vi "Teleop.vi"(10 "Match Info":T1={"Autonomous Elapsed Seconds"=0.0, "TeleOp Elapsed Seconds"=0.0, "Disabled Elapsed Seconds"=0.0, "Visited Autonomous"=FALSE, "Visited TeleOp"=FALSE, "Visited Disabled"=FALSE, "Autonomous Settings"={"Autonomous Style"=enum."Independent", "VI Refnum"=refnum}}, 11 "Call Context":T2) -> ()   [LabVIEW 2014]
doc: "This VI is called for each TeleOp packet received from the DS where the robot is not disabled. It is often used to read from the joysticks and update I/O or to update setpoints for timed control loops. It should complete and return within 20 milliseconds or it may miss DS packets."
uses:
  <vilib>/Rock Robotics/WPI/DriverStation/WPI_DriverStationDerivedRobotMode.ctl
  <vilib>/Rock Robotics/WPI/DriverStation/WPI_DriverStationMatch Info.ctl
  <vilib>/Rock Robotics/WPI/RobotDrive/WPI_RobotDriveGetSetRefNum.vi
  <vilib>/Rock Robotics/WPI/Joystick/WPI_JoystickGetSetRefNum.vi
  Robot Global Data.vi
  <vilib>/Rock Robotics/Network Tables/SD Write Boolean Array.vi
  <vilib>/Rock Robotics/Network Tables/SD Write Numeric Array.vi
  <vilib>/Rock Robotics/Network Tables/SD Read Number.vi
  <vilib>/Rock Robotics/Network Tables/SD Write Number.vi
  <vilib>/Rock Robotics/Network Tables/SD Write Boolean.vi
  <vilib>/Rock Robotics/WPI/RobotDrive/WPI_RobotDriveMecanumDrive_Cartesian.vi
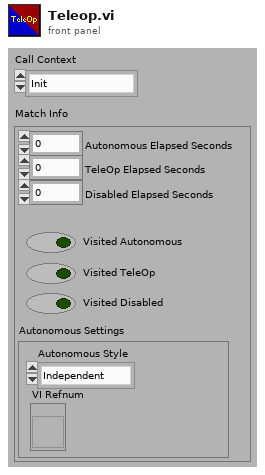
[diagram p1: front panel]
types:
  T1 = typedef "WPI_DriverStationMatch Info.ctl" = cluster{"Autonomous Elapsed Seconds":dbl, "TeleOp Elapsed Seconds":dbl, "Disabled Elapsed Seconds":dbl, "Visited Autonomous":bool, "Visited TeleOp":bool, "Visited Disabled":bool, "Autonomous Settings":cluster{"Autonomous Style":enum16{"Iterative", "Independent"}, "VI Refnum":refnum<vi>}}
  T2 = typedef "WPI_DriverStationDerivedRobotMode.ctl" = enum16{"Init", "Execute", "Stop"}
  T3 = typedef "WPI_RobotDriveDevRef.ctl" = cluster{"DevStatus":errorcluster, "Motors[]":T4[], "Square Inputs":bool, "Max Output":dbl}
  T4 = typedef "WPI_MotorControlDeviceRef.ctl" = cluster{"DeviceStatus":errorcluster, "Type":T5, "PWM":cluster{"Controller":T6, "PWM Channel":T7, "DeadBand":T8}, "CAN":cluster{"Device Number":u8, "Control Mode":T9, "Semaphore":T10, "Max Vout":dbl, "TalonSRX Control Mode":T11}, "Invert":bool, "TransformRef":T12, "InvTransformRef":T12}
  T5 = typedef "WPI_MotorControlType.ctl" = enum16{"PWM", "CAN", "CANTalonSRX"}
  T6 = typedef "FPGA_TypedefDigitalModule.ctl" = enum16{"Controller 1"}
  T7 = typedef "FPGA_DIOPWMChannel.ctl" = enum8{"PWM 0", "PWM 1", "PWM 2", "PWM 3", "PWM 4", "PWM 5", "PWM 6", "PWM 7", "PWM 8", "PWM 9", "PWM MXP 0", "PWM MXP 1", "PWM MXP 2", "PWM MXP 3", "PWM MXP 4", "PWM MXP 5", "PWM MXP 6", "PWM MXP 7", "PWM MXP 8", "PWM MXP 9", "Invalid"}
  T8 = typedef "WPI_PWMDeadband.ctl" = cluster{"Name":string, "maxPositivePwm":i32, "minPositivePwm":i32, "centerPwm":i32, "maxNegativePwm":i32, "minNegativePwm":i32, "angularRange":u16}
  T9 = typedef "WPI_CANJaguar_ControlMode.ctl" = enum8{"Percent VBus", "Current", "Speed", "Position", "Voltage"}
  T10 = typedef "Semaphore RefNum" = refnum<k1>
  T11 = typedef "WPI_CANTalonSRX_APIControlMode.ctl" = enum8{"Percent VBus", "Speed", "Position", "Slave", "Unchanged / Invalid"}
  T12 = typedef "WPI_PWMTransform_ConPane.ctl" = refnum<vi>
  T13 = typedef "WPI_JoystickDevRef.ctl" = cluster{"Device":T14}
  T14 = typedef "WPI_JoystickDeviceEnum.ctl" = enum16{"USB 0", "USB 1", "USB 2", "USB 3", "USB 4", "USB 5"}
  T15 = typedef "WPI_EncoderDevRef.ctl" = cluster{"DevStatus":errorcluster, "EncoderIndex":T16, "CounterIndex":T17, "DistancePerCount":dbl, "Decoding Type":T18}
  T16 = typedef "FPGA_EncoderIdx.ctl" = enum8{"Enc 0", "Enc 1", "Enc 2", "Enc 3", "Enc 4", "Enc 5", "Enc 6", "Enc 7", "Invalid"}
  T17 = typedef "FPGA_CounterCtrSystemIndex.ctl" = enum8{"Ctr 0", "Ctr 1", "Ctr 2", "Ctr 3", "Ctr 4", "Ctr 5", "Ctr 6", "Ctr 7", "Invalid"}
  T18 = typedef "WPI_EncoderType.ctl" = enum16{"1x", "2x", "4x"}
  T19 = typedef "WPI_GyroDevRef.ctl" = cluster{"DevStatus":errorcluster, "Analog Module":T20, "Analog Channel":T21, "Offset":dbl, "Gain (VoltsPerDegree/Second)":dbl}
  T20 = typedef "FPGA_TypedefAnalogModule.ctl" = enum16{"Controller 1"}
  T21 = typedef "FPGA_AIChannel.ctl" = enum8{"AI 0", "AI 1", "AI 2", "AI 3", "AI MXP 0", "AI MXP 1", "AI MXP 2", "AI MXP 3", "Invalid"}
  T22 = typedef "WPI_DigitalInputDevRef.ctl" = cluster{"DevStatus":errorcluster, "DIO Channel":T23, "Controller":T6}
  T23 = typedef "FPGA_DIOChannel.ctl" = enum8{"DIO 0", "DIO 1", "DIO 2", "DIO 3", "DIO 4", "DIO 5", "DIO 6", "DIO 7", "DIO 8", "DIO 9", "DIO MXP 0", "DIO MXP 1", "DIO MXP 2", "DIO MXP 3", "DIO MXP 4", "DIO MXP 5", "DIO MXP 6", "DIO MXP 7", "DIO MXP 8", "DIO MXP 9", "DIO MXP 10", "DIO MXP 11", "DIO MXP 12", "DIO MXP 13", "DIO MXP 14", "DIO MXP 15", "Invalid"}
  T24 = enum16{"Start", "Extending", "Lowering", "Grabbing", "Lifting", "Holding", "Placing", "Opening", "Dropping", "Score", "Exit", "Manual"}
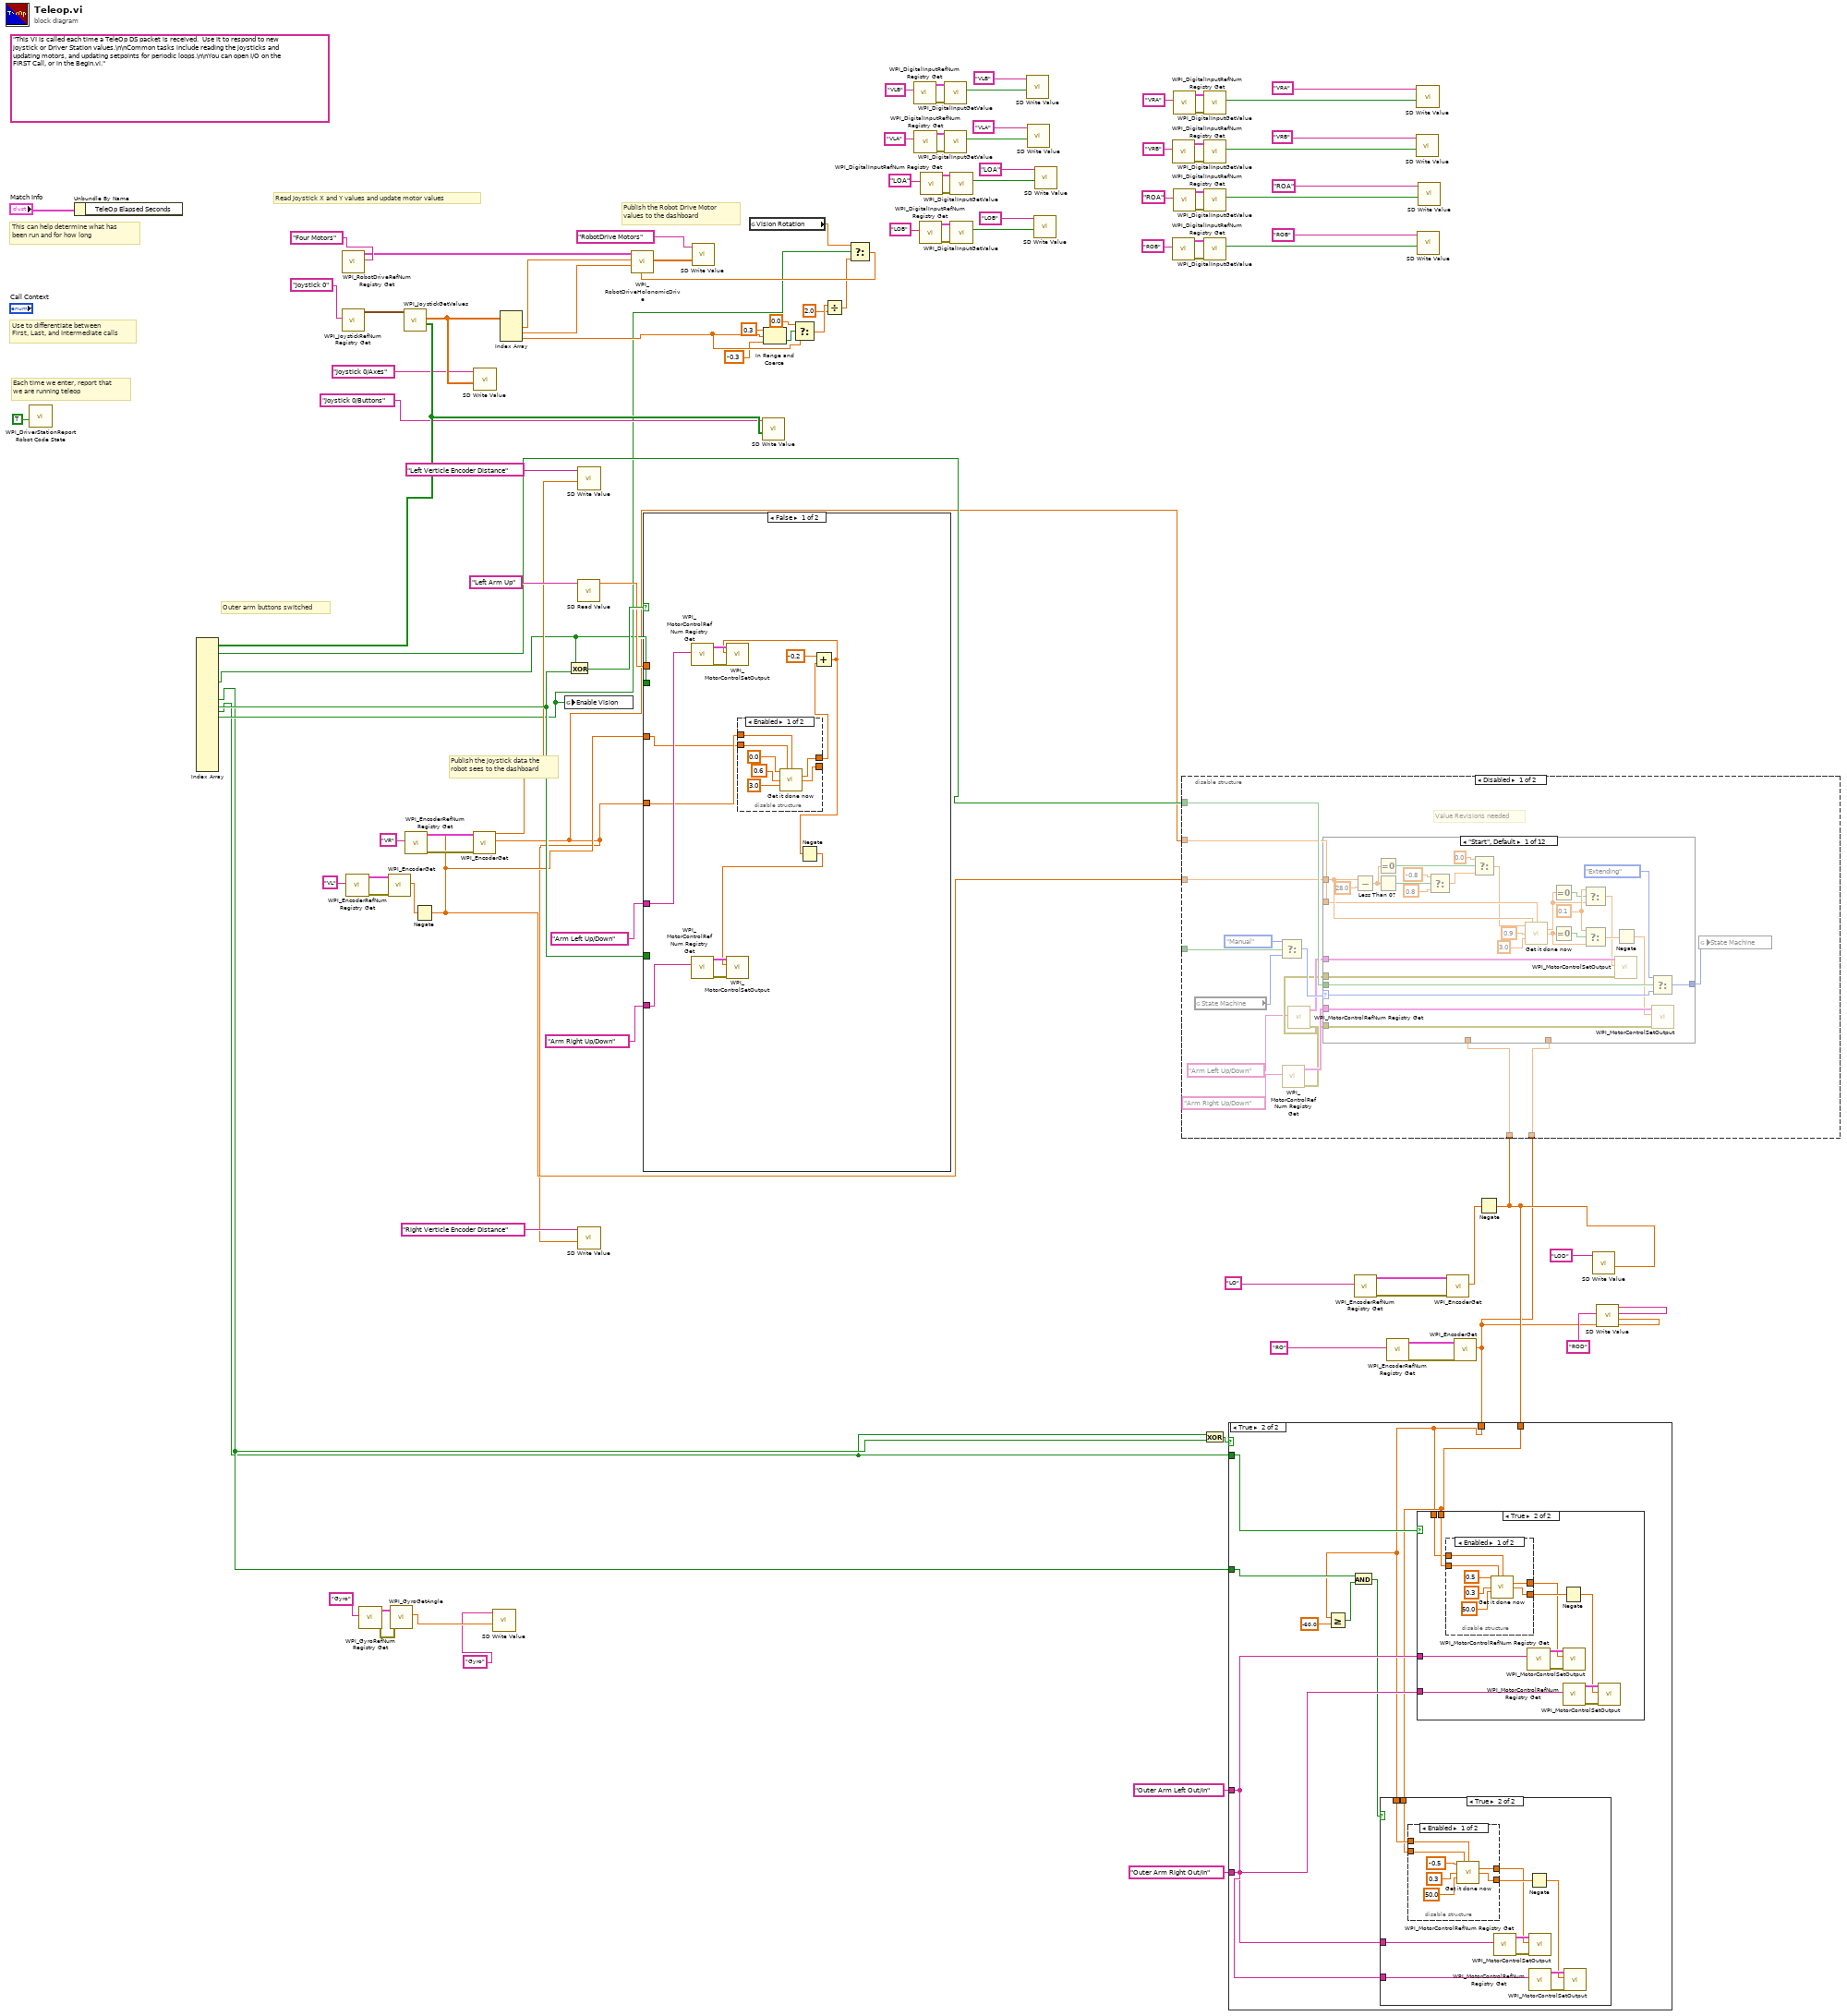
[diagram p0: block diagram]
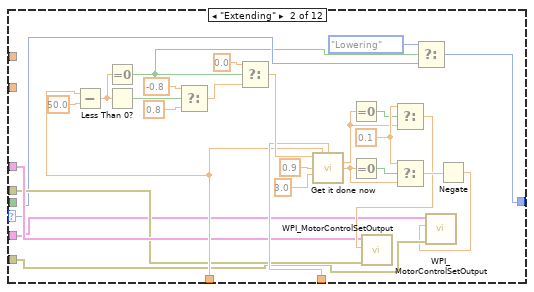
[diagram p2: hidden frame]
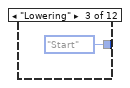
[diagram p3: hidden frame]
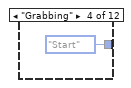
[diagram p4: hidden frame]
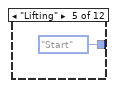
[diagram p5: hidden frame]
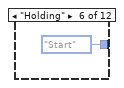
[diagram p6: hidden frame]
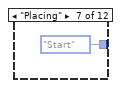
[diagram p7: hidden frame]
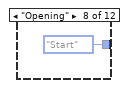
[diagram p8: hidden frame]
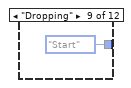
[diagram p9: hidden frame]
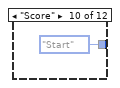
[diagram p10: hidden frame]
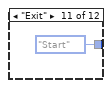
[diagram p11: hidden frame]
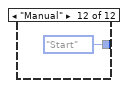
[diagram p12: hidden frame]
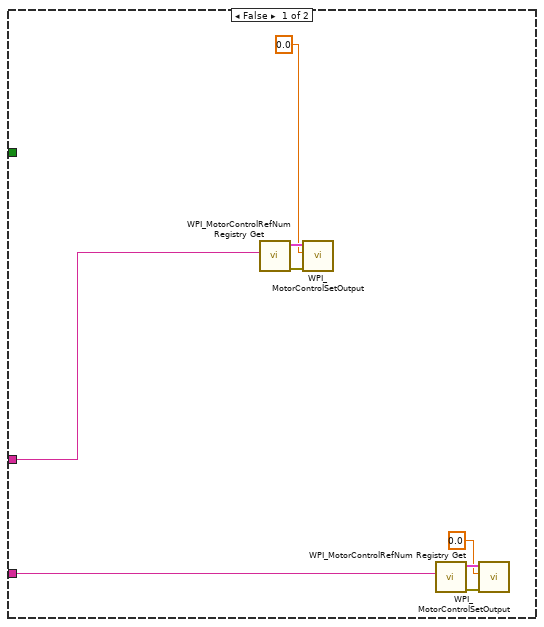
[diagram p14: hidden frame]
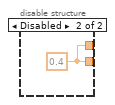
[diagram p16: hidden frame]
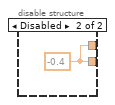
[diagram p18: hidden frame]
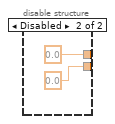
[diagram p19: hidden frame]
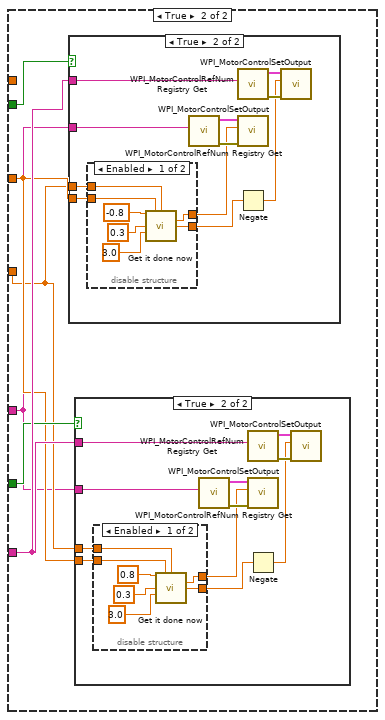
[diagram p20: hidden frame]
diagram:
  w6 = "ROD" ("Name")
  (unwired) "This VI is called each time a TeleOp DS packet is received.  Use it to respond to new joystick or Driver Station values.\n\nCommon tasks include reading the joysticks and updating motors, and updating setpoints for periodic loops.\n\nYou can open I/O on the FIRST Call, or in the Begin.vi."
  # "Outer arm buttons switched"
  # "Publish the joystick data the\nrobot sees to the dashboard"
  # "Publish the Robot Drive Motor\nvalues to the dashboard"
  # "Each time we enter, report that\nwe are running teleop"
  # "Use to differentiate between\nFirst, Last, and Intermediate calls"
  # "This can help determine what has\nbeen run and for how long"
  # "Read Joystick X and Y values and update motor values"
  n1 = call <vilib>:"WPI_DriverStationReport Robot Code State.vi"("TeleOp"=TRUE ("Autonomous")) -> ()  [unwired: 10 in, 1 out]
  n2 = Unbundle By Name("Match Info") -> ()  [unwired: 1 out]
  n3 = call <vilib>:"WPI_RobotDriveRefNum Registry Get.vi"("refnum name"="Four Motors") -> ("RobotDriveDevRef"=w103:T3)  [unwired: 1 in, 9 out]
  n4 = call <vilib>:"WPI_JoystickRefNum Registry Get.vi"("refnum name"="Joystick 0") -> ("JoystickDevRef"=w101:T13)  [unwired: 1 in, 9 out]
  n5 = call <vilib>:"WPI_EncoderRefNum Registry Get.vi"("refnum name"="VL") -> ("error out"=w80:errorcluster, "EncoderDevRef"=w81:T15)  [unwired: 9 in]
  n6 = call <vilib>:"WPI_GyroRefNum Registry Get.vi"("refnum name"="Gyro") -> ("error out"=w69:errorcluster, "GyroDevRef"=w68:T19)  [unwired: 9 in]
  n7 = call <vilib>:"WPI_EncoderGet.vi"("error in (no error)"=w80, "EncoderDevRef"=w81) -> ("Distance"=w62:dbl)  [unwired: 4 in, 5 out]
  n8 = call <vilib>:"WPI_GyroGetAngle.vi"("error in (no error)"=w69, "GyroDevRef"=w68) -> ("Angle"=w66:dbl)  [unwired: 6 in, 3 out]
  n9 = call <vilib>:"WPI_JoystickGetValues.vi"("JoystickDevRef"=w101) -> ("Buttons"=w96:bool[], "Axes"=w97:dbl[])  [unwired: 6 in, 3 out]
  n10 = Index Array(array=w96) -> (element #1=w11:bool, element #4=w90:bool, element #6=w8:bool, element #9=w4:bool, element #11=w3:bool, element #12=w9:bool)  [unwired: 21 in, 15 out]
  n11 = call <vilib>:"WPI_EncoderRefNum Registry Get.vi"("refnum name"="VR") -> ("error out"=w84:errorcluster, "EncoderDevRef"=w83:T15)  [unwired: 9 in]
  n12 = Negate(x=w62) -> (-x=w10:dbl)
  n13 = call <vilib>:"WPI_EncoderGet.vi"("error in (no error)"=w84, "EncoderDevRef"=w83) -> ("Distance"=w1:dbl)  [unwired: 4 in, 5 out]
  n14 = call-poly <vilib>:"SD Write Value.vi"("Numeric Array"=w97, "Name"="Joystick 0/Axes") -> ()  [unwired: 8 in, 2 out]
  n15 = call-poly <vilib>:"SD Write Value.vi"("Numeric"=w66, "Name"="Gyro") -> ()  [unwired: 8 in, 2 out]
  n16 = Index Array(array=w97) -> (element #1=w95:dbl, element #2=w94:dbl, element #3=w72:dbl)  [unwired: 3 in]
  n17 = global write "Robot Global Data.vi" "Enable Vision"(w9) -> ()
  n18 = Exclusive Or(1:w90, 2:w8) -> (0:w91:bool)
  n19 = call-poly <vilib>:"SD Read Value.vi"("Name"="Left Arm Up") -> ("Numeric"=w86:dbl)  [unwired: 8 in, 2 out]
  n20 = call-poly <vilib>:"SD Write Value.vi"("Numeric"=w10, "Name"="Left Verticle Encoder Distance") -> ()  [unwired: 8 in, 2 out]
  n21 = call-poly <vilib>:"SD Write Value.vi"("Numeric"=w1, "Name"="Right Verticle Encoder Distance") -> ()  [unwired: 8 in, 2 out]
  n22 = case shown="False" w91 {
    tunnel: w8 -> [_ w127]
    tunnel: w90 -> [_ w131]
    tunnel: "Arm Left Up/Down" ("refnum name") -> [w113 w128]
    tunnel: "Arm Right Up/Down" ("refnum name") -> [w112 w132]
    tunnel: w86 -> [_ _]
    tunnel: w1 -> [w111 w129]
    tunnel: w10 -> [w110 w130]
    frame False {
      n23 = call <vilib>:"WPI_MotorControlRefNum Registry Get.vi"("refnum name"=w113) -> ("error out"=w116:errorcluster, "MotorControlDevRef"=w117:T4)  [unwired: 9 in]
      n24 = call <vilib>:"WPI_MotorControlRefNum Registry Get.vi"("refnum name"=w112) -> ("error out"=w114:errorcluster, "MotorControlDevRef"=w115:T4)  [unwired: 9 in]
      n25 = disable-structure shown="Enabled" {
        disable-tunnel: w111 -> [w122 _]
        disable-tunnel: w110 -> [w121 _]
        disable-tunnel: [w123 0.0 ("Output")] -> _
        disable-tunnel: [w124 0.0 ("Output")] -> w109
        frame Enabled {
          n26 = call "Get it done now.vi"("Joystick Command"=0.0, "Encoder 0 Distance"=w121, "Encoder 1 Distance"=w122, "Maximum PWM Change"=0.6, "Max Following Error"=3.0) -> ("Motor 0 Command"=w124:dbl, "Motor 1 Command"=w123:dbl)  [unwired: 7 in, 2 out]
        }
        frame Disabled {
        }
      }
      n27 = Add(x=-0.2, y=w109) -> (x+y=w107:dbl)
      n28 = call <vilib>:"WPI_MotorControlSetOutput.vi"("error in (no error)"=w116, "Output"=w107, "MotorControlDevRef"=w117) -> ()  [unwired: 6 in, 3 out]
      n29 = Negate(x=w107) -> (-x=w106:dbl)
      n30 = call <vilib>:"WPI_MotorControlSetOutput.vi"("error in (no error)"=w114, "Output"=w106, "MotorControlDevRef"=w115) -> ()  [unwired: 6 in, 3 out]
    }
    frame True {
      n31 = case shown="True" w127 {
        tunnel: w128 -> [_ w139]
        tunnel: w132 -> [_ w133]
        tunnel: w129 -> [_ w138]
        tunnel: w130 -> [_ w137]
        frame False {
        }
        frame True {
          n32 = disable-structure shown="Enabled" {
            disable-tunnel: w138 -> [w150 _]
            disable-tunnel: w137 -> [w149 _]
            disable-tunnel: [w144 w151] -> w136
            disable-tunnel: [w145 w151] -> w134
            frame Enabled {
              n33 = call "Get it done now.vi"("Joystick Command"=-0.8 ("Maximum PWM Change"), "Encoder 0 Distance"=w149, "Encoder 1 Distance"=w150, "Maximum PWM Change"=0.3, "Max Following Error"=3.0) -> ("Motor 0 Command"=w145:dbl, "Motor 1 Command"=w144:dbl)  [unwired: 7 in, 2 out]
            }
            frame Disabled {
              w151 = 0.3 ("Motor 1 Command")
            }
          }
          n34 = call <vilib>:"WPI_MotorControlRefNum Registry Get.vi"("refnum name"=w139) -> ("error out"=w143:errorcluster, "MotorControlDevRef"=w142:T4)  [unwired: 9 in]
          n35 = call <vilib>:"WPI_MotorControlRefNum Registry Get.vi"("refnum name"=w133) -> ("error out"=w141:errorcluster, "MotorControlDevRef"=w140:T4)  [unwired: 9 in]
          n36 = call <vilib>:"WPI_MotorControlSetOutput.vi"("error in (no error)"=w143, "Output"=w134, "MotorControlDevRef"=w142) -> ()  [unwired: 6 in, 3 out]
          n37 = Negate(x=w136) -> (-x=w135:dbl)
          n38 = call <vilib>:"WPI_MotorControlSetOutput.vi"("error in (no error)"=w141, "Output"=w135, "MotorControlDevRef"=w140) -> ()  [unwired: 6 in, 3 out]
        }
      }
      n39 = case shown="True" w131 {
        tunnel: w128 -> [_ w158]
        tunnel: w132 -> [_ w157]
        tunnel: w130 -> [_ w156]
        tunnel: w129 -> [_ w155]
        frame False {
        }
        frame True {
          n40 = disable-structure shown="Enabled" {
            disable-tunnel: w156 -> [w166 _]
            disable-tunnel: w155 -> [w167 _]
            disable-tunnel: [w168 w170] -> w154
            disable-tunnel: [w169 w170] -> w152
            frame Enabled {
              n41 = call "Get it done now.vi"("Joystick Command"=0.8 ("Maximum PWM Change"), "Encoder 0 Distance"=w166, "Encoder 1 Distance"=w167, "Maximum PWM Change"=0.3, "Max Following Error"=3.0) -> ("Motor 0 Command"=w169:dbl, "Motor 1 Command"=w168:dbl)  [unwired: 7 in, 2 out]
            }
            frame Disabled {
              w170 = -0.3 ("Motor 1 Command")
            }
          }
          n42 = call <vilib>:"WPI_MotorControlRefNum Registry Get.vi"("refnum name"=w158) -> ("error out"=w162:errorcluster, "MotorControlDevRef"=w161:T4)  [unwired: 9 in]
          n43 = call <vilib>:"WPI_MotorControlRefNum Registry Get.vi"("refnum name"=w157) -> ("error out"=w160:errorcluster, "MotorControlDevRef"=w159:T4)  [unwired: 9 in]
          n44 = call <vilib>:"WPI_MotorControlSetOutput.vi"("error in (no error)"=w162, "Output"=w152, "MotorControlDevRef"=w161) -> ()  [unwired: 6 in, 3 out]
          n45 = Negate(x=w154) -> (-x=w153:dbl)
          n46 = call <vilib>:"WPI_MotorControlSetOutput.vi"("error in (no error)"=w160, "Output"=w153, "MotorControlDevRef"=w159) -> ()  [unwired: 6 in, 3 out]
        }
      }
    }
  }
  n47 = global read "Robot Global Data.vi" "Vision Rotation"() -> (w64:dbl)
  n48 = call-poly <vilib>:"SD Write Value.vi"("Boolean Array"=w96, "Name"="Joystick 0/Buttons") -> ()  [unwired: 8 in, 2 out]
  n49 = In Range and Coerce(upper limit=0.3, x=w72, lower limit=-0.3) -> (In Range?=w74:bool)  [unwired: 1 out]
  n50 = Select(t=0.0, s=w74, f=w72) -> (s? t:f=w14:dbl)
  n51 = Divide(x=w14, y=2.0) -> (x/y=w12:dbl)
  n52 = Select(t=w64, s=w9, f=w12) -> (s? t:f=w63:dbl)
  n53 = call-poly <vilib>:"WPI_RobotDriveHolonomicDrive.vi"("Rotation"=w63, "Y"=w94, "X"=w95, "RobotDriveDevRef"=w103) -> ("Motor Values"=w98:dbl[])  [unwired: 5 in, 2 out]
  n54 = call-poly <vilib>:"SD Write Value.vi"("Numeric Array"=w98, "Name"="RobotDrive Motors") -> ()  [unwired: 8 in, 2 out]
  n55 = call <vilib>:"WPI_DigitalInputRefNum Registry Get.vi"("refnum name"="VLB") -> ("error out"=w51:errorcluster, "DigitalInputDevRef"=w50:T22)  [unwired: 9 in]
  n56 = call <vilib>:"WPI_DigitalInputRefNum Registry Get.vi"("refnum name"="VLA") -> ("error out"=w53:errorcluster, "DigitalInputDevRef"=w52:T22)  [unwired: 9 in]
  n57 = call <vilib>:"WPI_DigitalInputRefNum Registry Get.vi"("refnum name"="LOB") -> ("error out"=w43:errorcluster, "DigitalInputDevRef"=w42:T22)  [unwired: 9 in]
  n58 = call <vilib>:"WPI_DigitalInputRefNum Registry Get.vi"("refnum name"="LOA") -> ("error out"=w45:errorcluster, "DigitalInputDevRef"=w44:T22)  [unwired: 9 in]
  n59 = call <vilib>:"WPI_DigitalInputGetValue.vi"("error in (no error)"=w51, "DigitalInputDevRef"=w50) -> ("Value"=w36:bool)  [unwired: 7 in, 2 out]
  n60 = call <vilib>:"WPI_DigitalInputGetValue.vi"("error in (no error)"=w53, "DigitalInputDevRef"=w52) -> ("Value"=w37:bool)  [unwired: 7 in, 2 out]
  n61 = call <vilib>:"WPI_DigitalInputGetValue.vi"("error in (no error)"=w45, "DigitalInputDevRef"=w44) -> ("Value"=w35:bool)  [unwired: 7 in, 2 out]
  n62 = call <vilib>:"WPI_DigitalInputGetValue.vi"("error in (no error)"=w43, "DigitalInputDevRef"=w42) -> ("Value"=w34:bool)  [unwired: 7 in, 2 out]
  n63 = call-poly <vilib>:"SD Write Value.vi"("Boolean"=w36, "Name"="VLB") -> ()  [unwired: 8 in, 2 out]
  n64 = call-poly <vilib>:"SD Write Value.vi"("Boolean"=w37, "Name"="VLA") -> ()  [unwired: 8 in, 2 out]
  n65 = call-poly <vilib>:"SD Write Value.vi"("Boolean"=w34, "Name"="LOB") -> ()  [unwired: 8 in, 2 out]
  n66 = call-poly <vilib>:"SD Write Value.vi"("Boolean"=w35, "Name"="LOA") -> ()  [unwired: 8 in, 2 out]
  n67 = call <vilib>:"WPI_DigitalInputRefNum Registry Get.vi"("refnum name"="VRB") -> ("error out"=w47:errorcluster, "DigitalInputDevRef"=w46:T22)  [unwired: 9 in]
  n68 = call <vilib>:"WPI_DigitalInputRefNum Registry Get.vi"("refnum name"="ROB") -> ("error out"=w41:errorcluster, "DigitalInputDevRef"=w40:T22)  [unwired: 9 in]
  n69 = call <vilib>:"WPI_DigitalInputRefNum Registry Get.vi"("refnum name"="VRA") -> ("error out"=w49:errorcluster, "DigitalInputDevRef"=w48:T22)  [unwired: 9 in]
  n70 = call <vilib>:"WPI_DigitalInputRefNum Registry Get.vi"("refnum name"="ROA") -> ("error out"=w39:errorcluster, "DigitalInputDevRef"=w38:T22)  [unwired: 9 in]
  n71 = call <vilib>:"WPI_DigitalInputGetValue.vi"("error in (no error)"=w49, "DigitalInputDevRef"=w48) -> ("Value"=w32:bool)  [unwired: 7 in, 2 out]
  n72 = call <vilib>:"WPI_DigitalInputGetValue.vi"("error in (no error)"=w47, "DigitalInputDevRef"=w46) -> ("Value"=w31:bool)  [unwired: 7 in, 2 out]
  n73 = call <vilib>:"WPI_DigitalInputGetValue.vi"("error in (no error)"=w39, "DigitalInputDevRef"=w38) -> ("Value"=w30:bool)  [unwired: 7 in, 2 out]
  n74 = call <vilib>:"WPI_DigitalInputGetValue.vi"("error in (no error)"=w41, "DigitalInputDevRef"=w40) -> ("Value"=w33:bool)  [unwired: 7 in, 2 out]
  n75 = Exclusive Or(1:w4, 2:w3) -> (0:w77:bool)
  n76 = call <vilib>:"WPI_EncoderRefNum Registry Get.vi"("refnum name"="LO") -> ("error out"=w19:errorcluster, "EncoderDevRef"=w21:T15)  [unwired: 9 in]
  n77 = call <vilib>:"WPI_EncoderRefNum Registry Get.vi"("refnum name"="RO") -> ("error out"=w18:errorcluster, "EncoderDevRef"=w16:T15)  [unwired: 9 in]
  n78 = call-poly <vilib>:"SD Write Value.vi"("Boolean"=w31, "Name"="VRB") -> ()  [unwired: 8 in, 2 out]
  n79 = call-poly <vilib>:"SD Write Value.vi"("Boolean"=w32, "Name"="VRA") -> ()  [unwired: 8 in, 2 out]
  n80 = call-poly <vilib>:"SD Write Value.vi"("Boolean"=w33, "Name"="ROB") -> ()  [unwired: 8 in, 2 out]
  n81 = call-poly <vilib>:"SD Write Value.vi"("Boolean"=w30, "Name"="ROA") -> ()  [unwired: 8 in, 2 out]
  n82 = call <vilib>:"WPI_EncoderGet.vi"("error in (no error)"=w19, "EncoderDevRef"=w21) -> ("Distance"=w15:dbl)  [unwired: 4 in, 5 out]
  n83 = call <vilib>:"WPI_EncoderGet.vi"("error in (no error)"=w18, "EncoderDevRef"=w16) -> ("Distance"=w2:dbl)  [unwired: 4 in, 5 out]
  n84 = Negate(x=w15) -> (-x=w7:dbl)
  n85 = disable-structure shown="Disabled" {
    disable-tunnel: _ -> [w183 _]
    disable-tunnel: w11 -> [w182 _]
    disable-tunnel: w1 -> [w180 _]
    disable-tunnel: w10 -> [w179 _]
    disable-tunnel: w7 -> [w172 _]
    disable-tunnel: w2 -> [w171 _]
    frame Disabled {
      # "Value Revisions needed"
      n86 = global read "Robot Global Data.vi" "State Machine"() -> (w186:T24)
      n87 = Select(t=T24."Manual", s=w183, f=w186) -> (s? t:f=w185:T24)
      n88 = call <vilib>:"WPI_MotorControlRefNum Registry Get.vi"("refnum name"="Arm Right Up/Down") -> ("error out"=w175:errorcluster, "MotorControlDevRef"=w176:T4)  [unwired: 9 in]
      n89 = call <vilib>:"WPI_MotorControlRefNum Registry Get.vi"("refnum name"="Arm Left Up/Down") -> ("error out"=w177:errorcluster, "MotorControlDevRef"=w178:T4)  [unwired: 9 in]
      n90 = case shown="\"Start\", Default" w185 {
        selector: w185 -> [w214 w218 _ _ _ _ _ _ _ _ _ _]
        tunnel: w182 -> [w215 _ _ _ _ _ _ _ _ _ _ _]
        tunnel: [w213 w219 T24."Start" ("State Machine") T24."Start" ("State Machine") T24."Start" ("State Machine") T24."Start" ("State Machine") T24."Start" ("State Machine") T24."Start" ("State Machine") T24."Start" ("State Machine") T24."Start" ("State Machine") T24."Start" ("State Machine") T24."Start" ("State Machine")] -> w181
        tunnel: w180 -> [w200 _ _ _ _ _ _ _ _ _ _ _]
        tunnel: w179 -> [w201 _ _ _ _ _ _ _ _ _ _ _]
        tunnel: w178 -> [w211 w224 _ _ _ _ _ _ _ _ _ _]
        tunnel: w177 -> [w210 w223 _ _ _ _ _ _ _ _ _ _]
        tunnel: w176 -> [w208 w222 _ _ _ _ _ _ _ _ _ _]
        tunnel: w175 -> [w207 w221 _ _ _ _ _ _ _ _ _ _]
        tunnel: w172 -> [_ w226 _ _ _ _ _ _ _ _ _ _]
        tunnel: w171 -> [_ w227 _ _ _ _ _ _ _ _ _ _]
        frame "Start", Default {
          w190 = 0.1 ("t")
          n91 = Subtract(x=w201, y=28.0) -> (x-y=w195:dbl)
          n92 = Equal To 0?(x=w195) -> (x = 0?=w198:bool)
          n93 = Less Than 0?(x=w195) -> (x < 0?=w206:bool)
          n94 = Select(t=-0.8, s=w206, f=0.8) -> (s? t:f=w199:dbl)
          n95 = Select(t=0.0, s=w198, f=w199) -> (s? t:f=w196:dbl)
          n96 = call "Get it done now.vi"("Joystick Command"=w196, "Encoder 0 Distance"=w201, "Encoder 1 Distance"=w200, "Maximum PWM Change"=0.9, "Max Following Error"=3.0) -> ("Motor 0 Command"=w188:dbl, "Motor 1 Command"=w193:dbl)  [unwired: 7 in, 2 out]
          n97 = Equal To 0?(x=w188) -> (x = 0?=w189:bool)
          n98 = Equal To 0?(x=w193) -> (x = 0?=w192:bool)
          n99 = Select(t=w190, s=w189, f=w188) -> (s? t:f=w187:dbl)
          n100 = Select(t=w190, s=w192, f=w193) -> (s? t:f=w191:dbl)
          n101 = call <vilib>:"WPI_MotorControlSetOutput.vi"("error in (no error)"=w210, "Output"=w187, "MotorControlDevRef"=w211) -> ()  [unwired: 6 in, 3 out]
          n102 = Negate(x=w191) -> (-x=w194:dbl)
          n103 = Select(t=T24."Extending", s=w215, f=w214) -> (s? t:f=w213:T24)
          n104 = call <vilib>:"WPI_MotorControlSetOutput.vi"("error in (no error)"=w207, "Output"=w194, "MotorControlDevRef"=w208) -> ()  [unwired: 6 in, 3 out]
        }
        frame "Extending" {
          w230 = 0.1 ("t")
          n105 = Subtract(x=w226, y=50.0) -> (x-y=w234:dbl)
          n106 = Equal To 0?(x=w234) -> (x = 0?=w217:bool)
          n107 = Less Than 0?(x=w234) -> (x < 0?=w242:bool)
          n108 = Select(t=-0.8, s=w242, f=0.8) -> (s? t:f=w237:dbl)
          n109 = Select(t=0.0, s=w217, f=w237) -> (s? t:f=w235:dbl)
          n110 = call "Get it done now.vi"("Joystick Command"=w235, "Encoder 0 Distance"=w226, "Encoder 1 Distance"=w227, "Maximum PWM Change"=0.9, "Max Following Error"=3.0) -> ("Motor 0 Command"=w228:dbl, "Motor 1 Command"=w233:dbl)  [unwired: 7 in, 2 out]
          n111 = Equal To 0?(x=w228) -> (x = 0?=w229:bool)
          n112 = Equal To 0?(x=w233) -> (x = 0?=w232:bool)
          n113 = Select(t=w230, s=w229, f=w228) -> (s? t:f=w225:dbl)
          n114 = call <vilib>:"WPI_MotorControlSetOutput.vi"("error in (no error)"=w223, "Output"=w225, "MotorControlDevRef"=w224) -> ()  [unwired: 6 in, 3 out]
          n115 = Select(t=w230, s=w232, f=w233) -> (s? t:f=w231:dbl)
          n116 = Select(t=T24."Lowering", s=w217, f=w218) -> (s? t:f=w219:T24)
          n117 = Negate(x=w231) -> (-x=w220:dbl)
          n118 = call <vilib>:"WPI_MotorControlSetOutput.vi"("error in (no error)"=w221, "Output"=w220, "MotorControlDevRef"=w222) -> ()  [unwired: 6 in, 3 out]
        }
        frame "Lowering" {
        }
        frame "Grabbing" {
        }
        frame "Lifting" {
        }
        frame "Holding" {
        }
        frame "Placing" {
        }
        frame "Opening" {
        }
        frame "Dropping" {
        }
        frame "Score" {
        }
        frame "Exit" {
        }
        frame "Manual" {
        }
      }
      n119 = global write "Robot Global Data.vi" "State Machine"(w181) -> ()
    }
    frame Enabled {
    }
  }
  n120 = case shown="True" w77 {
    tunnel: w4 -> [_ w266]
    tunnel: w3 -> [_ w270]
    tunnel: "Outer Arm Right Out/In" ("refnum name") -> [w256 w269]
    tunnel: "Outer Arm Left Out/In" ("refnum name") -> [w255 w268]
    tunnel: w7 -> [_ w267]
    tunnel: w2 -> [_ w263]
    frame False {
      n121 = call <vilib>:"WPI_MotorControlRefNum Registry Get.vi"("refnum name"=w255) -> ("error out"=w258:errorcluster, "MotorControlDevRef"=w259:T4)  [unwired: 9 in]
      n122 = call <vilib>:"WPI_MotorControlSetOutput.vi"("error in (no error)"=w258, "Output"=0.0, "MotorControlDevRef"=w259) -> ()  [unwired: 6 in, 3 out]
      n123 = call <vilib>:"WPI_MotorControlRefNum Registry Get.vi"("refnum name"=w256) -> ("error out"=w260:errorcluster, "MotorControlDevRef"=w261:T4)  [unwired: 9 in]
      n124 = call <vilib>:"WPI_MotorControlSetOutput.vi"("error in (no error)"=w260, "Output"=0.0, "MotorControlDevRef"=w261) -> ()  [unwired: 6 in, 3 out]
    }
    frame True {
      n125 = Greater Or Equal?(x=w263, y=-60.0) -> (x >= y?=w262:bool)
      n126 = And(x=w266, y=w262) -> (x .and. y?=w265:bool)
      n127 = case shown="True" w265 {
        tunnel: w269 -> [_ w296]
        tunnel: w268 -> [_ w295]
        tunnel: w263 -> [_ w291]
        tunnel: w267 -> [_ w290]
        frame False {
        }
        frame True {
          n128 = disable-structure shown="Enabled" {
            disable-tunnel: [w304 w308] -> w294
            disable-tunnel: [w303 w308] -> w292
            disable-tunnel: w291 -> [w302 _]
            disable-tunnel: w290 -> [w301 _]
            frame Enabled {
              n129 = call "Get it done now.vi"("Joystick Command"=-0.5, "Encoder 0 Distance"=w301, "Encoder 1 Distance"=w302, "Maximum PWM Change"=0.3, "Max Following Error"=50.0) -> ("Motor 0 Command"=w303:dbl, "Motor 1 Command"=w304:dbl)  [unwired: 7 in, 2 out]
            }
            frame Disabled {
              w308 = -0.4 ("Output")
            }
          }
          n130 = call <vilib>:"WPI_MotorControlRefNum Registry Get.vi"("refnum name"=w295) -> ("error out"=w298:errorcluster, "MotorControlDevRef"=w297:T4)  [unwired: 9 in]
          n131 = Negate(x=w294) -> (-x=w293:dbl)
          n132 = call <vilib>:"WPI_MotorControlSetOutput.vi"("error in (no error)"=w298, "Output"=w292, "MotorControlDevRef"=w297) -> ()  [unwired: 6 in, 3 out]
          n133 = call <vilib>:"WPI_MotorControlRefNum Registry Get.vi"("refnum name"=w296) -> ("error out"=w300:errorcluster, "MotorControlDevRef"=w299:T4)  [unwired: 9 in]
          n134 = call <vilib>:"WPI_MotorControlSetOutput.vi"("error in (no error)"=w300, "Output"=w293, "MotorControlDevRef"=w299) -> ()  [unwired: 6 in, 3 out]
        }
      }
      n135 = case shown="True" w270 {
        tunnel: w269 -> [_ w277]
        tunnel: w268 -> [_ w276]
        tunnel: w267 -> [_ w275]
        tunnel: w263 -> [_ w274]
        frame False {
        }
        frame True {
          n136 = disable-structure shown="Enabled" {
            disable-tunnel: w275 -> [w288 _]
            disable-tunnel: w274 -> [w287 _]
            disable-tunnel: [w282 w289] -> w273
            disable-tunnel: [w283 w289] -> w271
            frame Enabled {
              n137 = call "Get it done now.vi"("Joystick Command"=0.5, "Encoder 0 Distance"=w288, "Encoder 1 Distance"=w287, "Maximum PWM Change"=0.3, "Max Following Error"=50.0) -> ("Motor 0 Command"=w283:dbl, "Motor 1 Command"=w282:dbl)  [unwired: 7 in, 2 out]
            }
            frame Disabled {
              w289 = 0.4 ("Motor 1 Command")
            }
          }
          n138 = call <vilib>:"WPI_MotorControlRefNum Registry Get.vi"("refnum name"=w276) -> ("error out"=w279:errorcluster, "MotorControlDevRef"=w278:T4)  [unwired: 9 in]
          n139 = Negate(x=w273) -> (-x=w272:dbl)
          n140 = call <vilib>:"WPI_MotorControlSetOutput.vi"("error in (no error)"=w279, "Output"=w271, "MotorControlDevRef"=w278) -> ()  [unwired: 6 in, 3 out]
          n141 = call <vilib>:"WPI_MotorControlRefNum Registry Get.vi"("refnum name"=w277) -> ("error out"=w281:errorcluster, "MotorControlDevRef"=w280:T4)  [unwired: 9 in]
          n142 = call <vilib>:"WPI_MotorControlSetOutput.vi"("error in (no error)"=w281, "Output"=w272, "MotorControlDevRef"=w280) -> ()  [unwired: 6 in, 3 out]
        }
      }
    }
  }
  n143 = call-poly <vilib>:"SD Write Value.vi"("Numeric"=w7, "Name"="LOD") -> ()  [unwired: 8 in, 2 out]
  n144 = call-poly <vilib>:"SD Write Value.vi"("Numeric"=w2, "Table Prefix"=w6, "Name"=w6) -> ()  [unwired: 7 in, 2 out]
